vi "lsl destroy outlet.vi"(8 "error in (no error)":errorcluster, 11 "outlet":T1) -> (0 "error out":errorcluster)   [LabVIEW 2019, in "Lab Streaming Layer.lvlib"]
doc: "extern LIBLSL_C_API void lsl_destroy_outlet(lsl_outlet out);"
uses:
  Lab Streaming Layer.lvlib
  Custom Controls/lsl_outlet.ctl
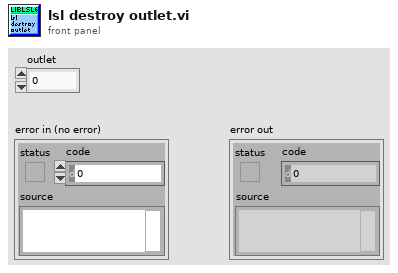
[diagram p1: front panel]
types:
  T1 = typedef "Lab Streaming Layer.lvlib/lsl_outlet.ctl" = u64
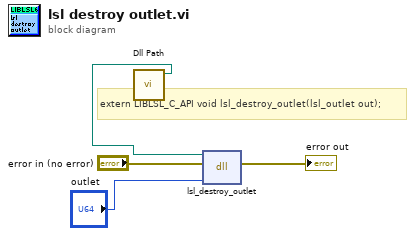
[diagram p0: block diagram]
diagram:
  # "extern LIBLSL_C_API void lsl_destroy_outlet(lsl_outlet out);"
  n1 = call "Dll Path.vi"() -> ("Dll path"=w1:path)  [unwired: 11 in]
  n2 = dll-call lib="E:/LabStreamingLayer/liblsl-LabVIEW-master/liblsl-LabVIEW-master/lsl.dll" fn="lsl_destroy_outlet"(path in=w1, error in="error in (no error)", "out"="outlet") -> (error out=→"error out":errorcluster)  [unwired: 3 in, 1 out]
